vi "IV-curve-2.vi"() -> ()   [LabVIEW 2012]
uses:
  <instrlib>/Tektronix PWS4XXX Series/Tektronix PWS4XXX Series.lvlib
panel:
  in  "Clean plot":bool
  in  "True voltage":bool=TRUE
  in  "Delay V(in) / I(out) (ms)":u32=100
  in  "Tab Control":T1(tab)
  in  "Start":bool
  out "Voltage-Current Curve":cluster{dbl[], dbl[]}[](graph)
  in  "Stop":bool
  in  "Umax, V":dbl=2.0
  in  "Umin, V":dbl
  in  "Step":dbl=0.2
  in  "Imax (0-3A)":dbl=0.1 format="%.2f"
  out "Current, A":dbl
  out "Voltage, V":dbl
  out "Time, s":dbl format="%#.1g"
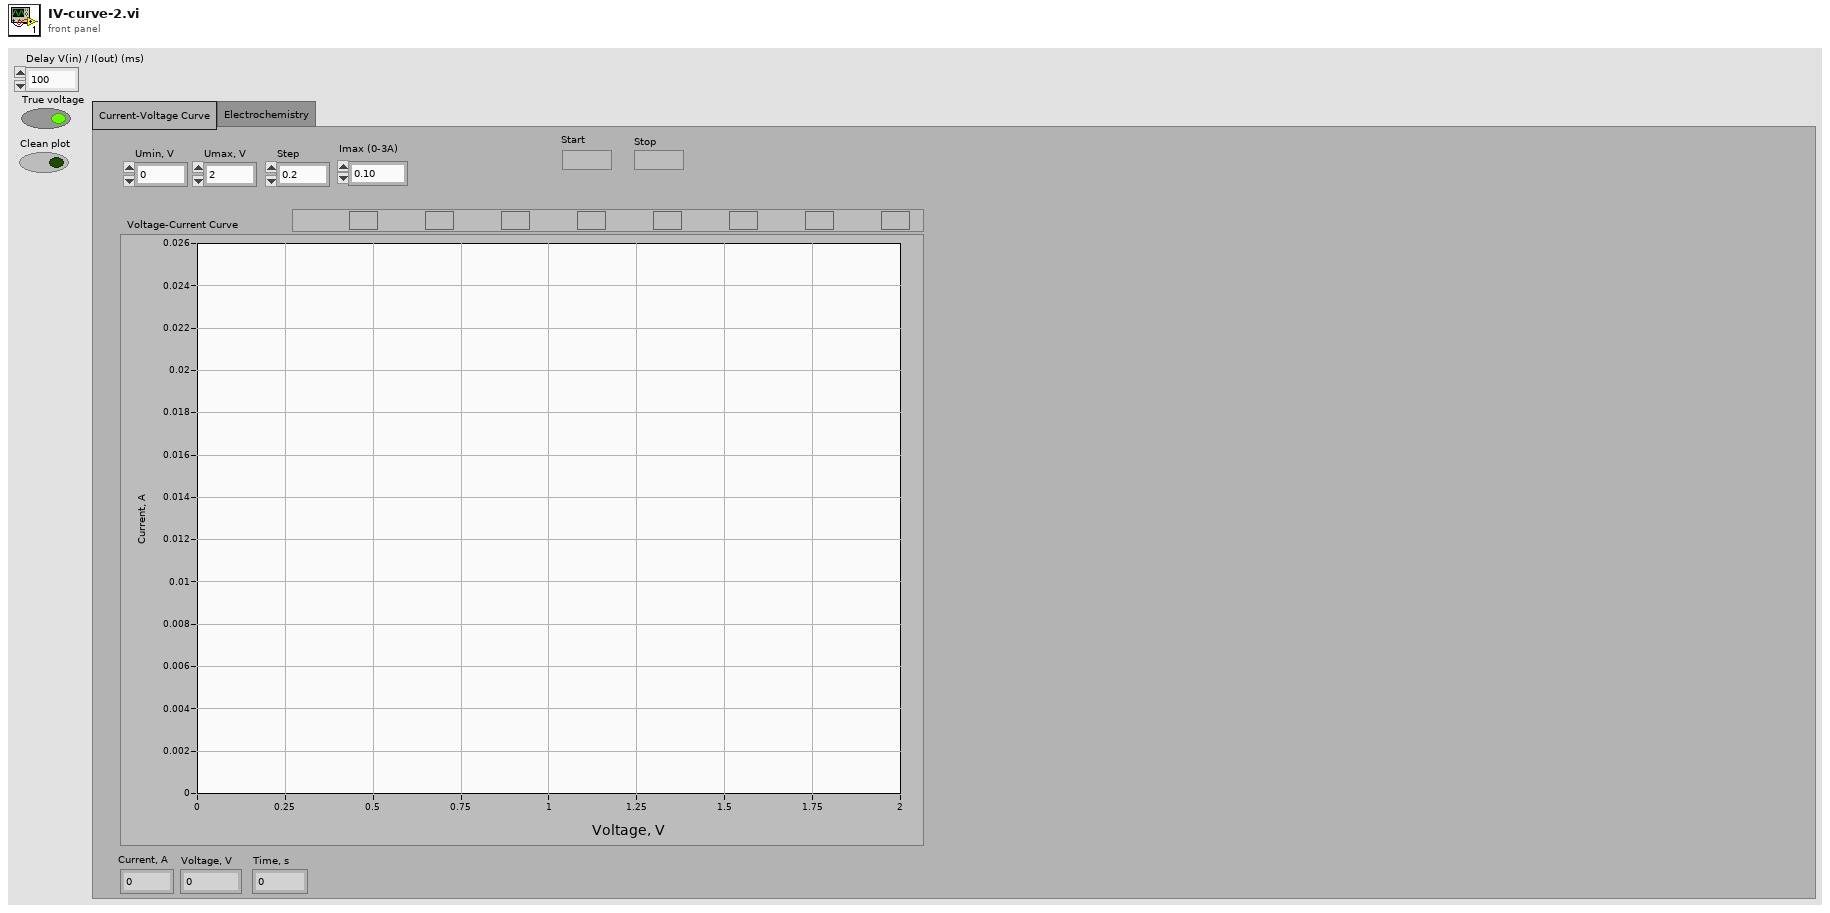
[diagram p1: front panel]
types:
  T1 = enum32{"Current-Voltage Curve", "Electrochemistry"}
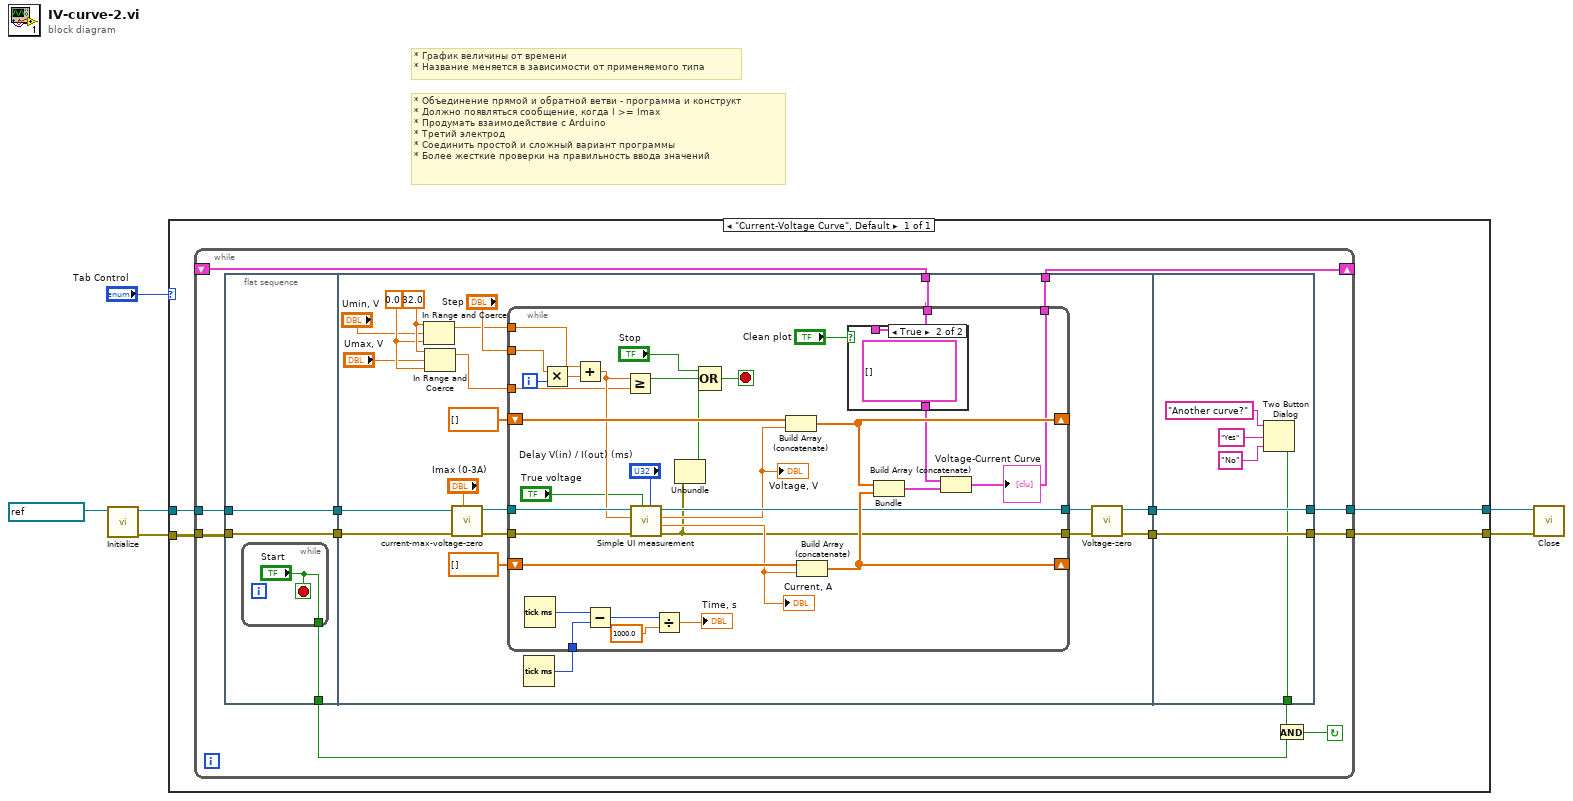
[diagram p0: block diagram]
diagram:
  # "* Объединение прямой и обратной ветви - программа и конструкт\n* Должно появляться сообщение, когда I >= Imax\n* Продумать взаимодействие с Arduino\n* Третий электрод\n* Соединить простой и сложный вариант программы\n* Более жесткие проверки на правильность ввода значений"
  # "* График величины от времени\n* Название меняется в зависимости от применяемого типа"
  n1 = call <instrlib>:"Initialize.vi"("VISA resource name"=refnum<visa-resource-name> "PWS4323") -> ("error out"=w4:errorcluster, "VISA resource name out"=w5:refnum<visa-resource-name>)  [unwired: 9 in]
  n2 = case shown="\"Current-Voltage Curve\", Default" "Tab Control" {
    tunnel: w5 -> [w10]
    tunnel: w4 -> [w9]
    tunnel: [w8] -> w2
    tunnel: [w7] -> w1
    frame "Current-Voltage Curve", Default {
      n3 = while {
        tunnel: w10 -> [w23]
        tunnel: w9 -> [w22]
        tunnel: [w21] -> w8
        tunnel: [w20] -> w7
        shift-right: [w19] -> _
        shift-left: _ -> [w18]
        stop <- w14 continue-if-true
        n4 = flat-sequence {
          tunnel: w22 -> [w25]
          tunnel: w23 -> [w26]
          tunnel: [w26] -> w13
          tunnel: [w25] -> w12
          tunnel: [w24] -> w11
          tunnel: [w38] -> w19
          tunnel: w18 -> [w37]
          tunnel: [w46] -> w17
          tunnel: [w45] -> w16
          tunnel: w12 -> [w47]
          tunnel: w13 -> [w48]
          tunnel: [w87] -> w20
          tunnel: [w88] -> w21
          tunnel: w17 -> [w88]
          tunnel: w16 -> [w87]
          tunnel: [w83] -> w15
          frame #0 {
            n5 = while {
              tunnel: ["Start"] -> w24
              stop <- "Start" stop-if-true
            }
          }
          frame #1 {
            w31 = 0.0 ("lower limit")
            w32 = 32.0 ("upper limit")
            n6 = In Range and Coerce(upper limit=w32, x="Umin, V", lower limit=w31) -> (coerced(x)=w34:dbl)  [unwired: 1 out]
            n7 = In Range and Coerce(upper limit=w32, x="Umax, V", lower limit=w31) -> (coerced(x)=w33:dbl)  [unwired: 1 out]
            n8 = call "current-max-voltage-zero.vi"("Imax (0-3A)"="Imax (0-3A)", "error in (no error)"=w47, "VISA resource"=w48) -> ("error out"=w42:errorcluster, "VISA resource name out"=w43:refnum<visa-resource-name>)  [unwired: 6 in]
            n9 = Tick Count (ms)() -> (millisecond timer value=w28:u32)
            n10 = while {
              shift-right: [w75] -> _
              shift-left: dbl[] [] -> [w76]
              shift-right: [w79] -> _
              shift-left: dbl[] [] -> [w80]
              tunnel: [w69] -> w40
              tunnel: [w66] -> w39
              tunnel: w43 -> [w74]
              tunnel: w42 -> [w73]
              tunnel: [w61] -> w38
              tunnel: w37 -> [w59]
              tunnel: "Step" -> [w56]
              tunnel: w34 -> [w55]
              tunnel: w33 -> [w54]
              tunnel: w28 -> [w53]
              i -> [w78]
              stop <- w63 stop-if-true
              n11 = Tick Count (ms)() -> (millisecond timer value=w52:u32)
              n12 = Multiply(x=w56, y=w78) -> (x*y=w77:dbl)
              n13 = Add(x=w55, y=w77) -> (x+y=w72:dbl)
              n14 = Subtract(x=w52, y=w53) -> (x-y=w51:u32)
              n15 = Greater Or Equal?(x=w72, y=w54) -> (x >= y?=w64:bool)
              n16 = call "Simple UI measurement.vi"("Delay between V(in) and I(out) (ms)"="Delay V(in) / I(out) (ms)", "True voltage"="True voltage", "error in"=w73, "Voltage in, V"=w72, "VISA resource in"=w74) -> ("error out"=w66:errorcluster, "Current, A"=w67:dbl, "Voltage out, V"=w68:dbl, "VISA resource out"=w69:refnum<visa-resource-name>)  [unwired: 3 in]
              "Current, A" <- w67
              "Voltage, V" <- w68
              n17 = Divide(x=w51, y=1000.0) -> (x/y=→"Time, s":dbl)
              n18 = Unbundle(w66) -> ("status"=w65:bool)  [unwired: 2 out]
              n19 = Compound Arithmetic op=OR("Stop", w64, w65) -> (w63:bool)
              n20 = Build Array (concatenate)(w76, w68) -> (w75:dbl[])
              n21 = Build Array (concatenate)(w80, w67) -> (w79:dbl[])
              n22 = case shown="True" "Clean plot" {
                tunnel: w59 -> [w81 _]
                tunnel: [w81 cluster{dbl[], dbl[]}[] [] ("array")] -> w57
                frame False {
                }
                frame True {
                }
              }
              n23 = Bundle(w75, w79) -> (w62:cluster{dbl[], dbl[]})  [unwired: 1 in]
              n24 = Build Array (concatenate)(w57, w62) -> (w61:cluster{dbl[], dbl[]}[])
              "Voltage-Current Curve" <- w61
            }
            n25 = call "Voltage-zero.vi"("error in"=w39, "VISA resource in"=w40) -> ("error out"=w45:errorcluster, "VISA resource out"=w46:refnum<visa-resource-name>)  [unwired: 8 in]
          }
          frame #2 {
            n26 = Two Button Dialog(message="Another curve?", 1:"No" ("F button name (\"Cancel\")"), 2:"Yes" ("T button name (\"OK\")")) -> (T button?=w83:bool)
          }
        }
        n27 = And(x=w15, y=w11) -> (x .and. y?=w14:bool)
      }
    }
  }
  n28 = call <instrlib>:"Close.vi"("error in (no error)"=w1, "VISA resource name"=w2) -> ()  [unwired: 9 in, 1 out]
